vi "InclinometerCheckForTimeout.vi"(11 "InclinometerSampleSensorLoopData in":T1) -> (3 "InclinometerSampleSensorLoopData out":T1)   [LabVIEW 2016]
uses:
  InclinometerSampleSensorLoopData.ctl
  InclinometerSampleSensorLoopStates.ctl
  InclinometerSample.ctl
  InclinometerErrorSample.ctl
  InclinometerErrorCodes.ctl
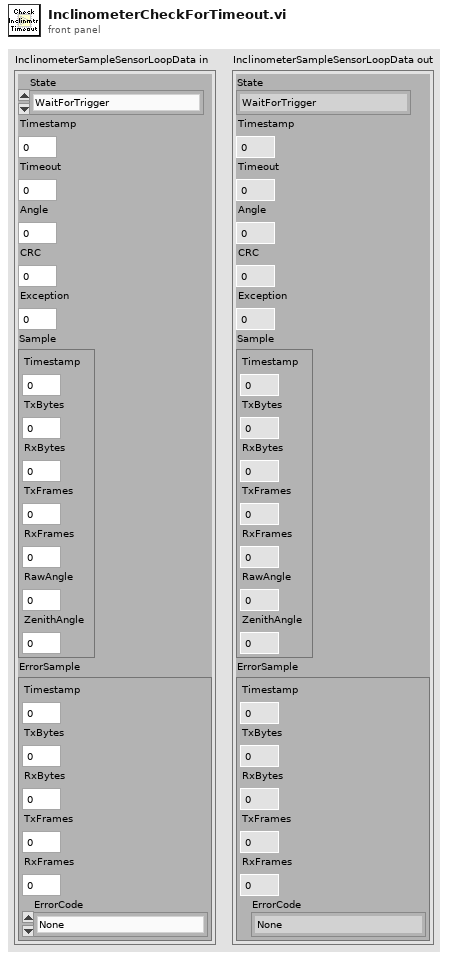
[diagram p1: front panel]
types:
  T1 = typedef "InclinometerSampleSensorLoopData.ctl" = cluster{"State":T2, "Timestamp":u64, "Timeout":i32, "Angle":u32, "CRC":u16, "Exception":u8, "Sample":T3, "ErrorSample":T4}
  T2 = typedef "InclinometerSampleSensorLoopStates.ctl" = enum16{"WaitForTrigger", "ClearRxFIFO", "WaitForClearComplete", "WriteAddress", "WriteFunction", "WriteStartAddress1", "WriteStartAddress0", "WriteAddressCount1", "WriteAddressCount0", "WriteCRC1", "WriteCRC0", "ReadAddress", "ReadFunction", "ReadByteCount", "ReadDataByte1", "ReadDataByte0", "ReadDataByte3", "ReadDataByte2", "ReadCRCByte0", "ReadCRCByte1", "CalculateCRC", "ValidateCRC", "PrepareSample", "MoveSample", "ReadExceptionCode", "ReadExceptionCRCByte0", "ReadExceptionCRCByte1", "CalculateExceptionCRC", "ValidateExceptionCRC", "ParseExceptionCode", "ResponseAddressError", "ResponseFunctionCodeError", "ResponseByteCountError", "ResponseCRCError", "ResponseUnknownError", "ResponseTimeoutError", "SensorReportsIllegalFunction", "SensorReportsIllegalDataAddress", "PrepareErrorCode", "MoveErrorCode"}
  T3 = typedef "InclinometerSample.ctl" = cluster{"Timestamp":u64, "TxBytes":u64, "RxBytes":u64, "TxFrames":u64, "RxFrames":u64, "RawAngle":i32, "ZenithAngle":sgl}
  T4 = typedef "InclinometerErrorSample.ctl" = cluster{"Timestamp":u64, "TxBytes":u64, "RxBytes":u64, "TxFrames":u64, "RxFrames":u64, "ErrorCode":T5}
  T5 = typedef "InclinometerErrorCodes.ctl" = enum8{"None", "ResponseAddressError", "ResponseFunctionCodeError", "ResponseByteCountError", "ResponseCRCError", "ResponseUnknownError", "ResponseTimeoutError", "SensorReportsIllegalFunction", "SensorReportsIllegalDataAddress"}
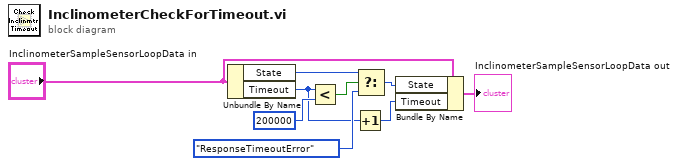
[diagram p0: block diagram]
diagram:
  n1 = Unbundle By Name("InclinometerSampleSensorLoopData in") -> ("State"=w1:T2, "Timeout"=w4:i32)
  n2 = Less?(x=w4, y=200000) -> (x < y?=w7:bool)
  n3 = Increment(x=w4) -> (x+1=w9:i32)
  n4 = Select(t=w1, s=w7, f=InclinometerSampleSensorLoopStates."ResponseTimeoutError" ("InclinometerState")) -> (s? t:f=w5:T2)
  n5 = Bundle By Name(cluster="InclinometerSampleSensorLoopData in", "State"=w5, "Timeout"=w9) -> (→"InclinometerSampleSensorLoopData out":T1)
